vi "GetCommand.vi"(8 "error in (no error)":errorcluster, 11 "Controller in":refnum<class "Controller.lvclass">) -> (0 "error out":errorcluster, 3 "Controller out":refnum<class "Controller.lvclass">)   [LabVIEW 2014, in "Controller.lvclass"]
uses:
  Controller.lvclass
  <vilib>/Utility/inputDevices.llb/joystickAcquire.vi
panel:
  in  "DeviceType":refnum<k1>
  out "DeviceType":refnum<k1>
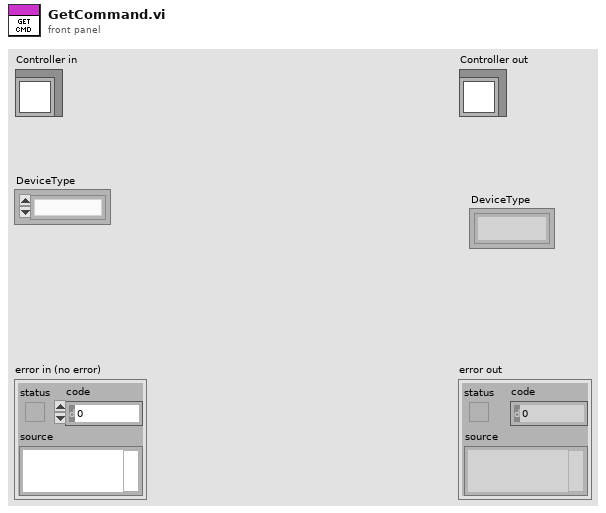
[diagram p1: front panel]
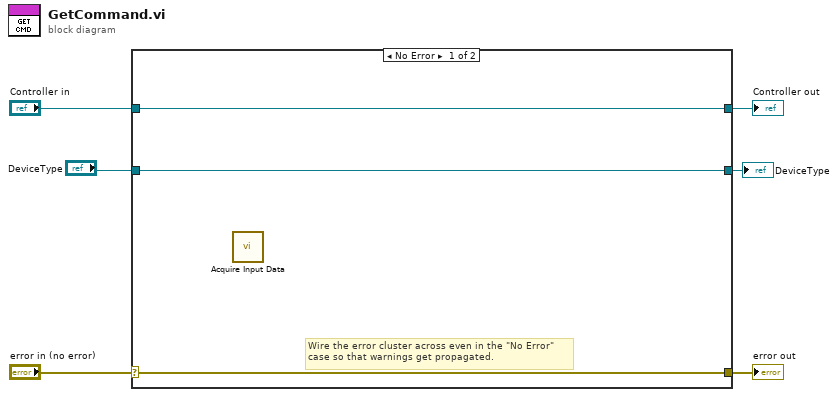
[diagram p0: block diagram]
diagram:
  n1 = case shown="No Error" "error in (no error)" {
    selector: "error in (no error)" -> [w8 w11]
    tunnel: [w8 w11] -> w5
    tunnel: [w9 w10] -> w3
    tunnel: "Controller in" -> [w9 w10]
    tunnel: "DeviceType" -> [w7 _]
    tunnel: [w7 _] -> w1
    frame No Error {
      # "Wire the error cluster across even in the \"No Error\"\ncase so that warnings get propagated."
      n2 = call-poly <vilib>:"Acquire Input Data.vi"() -> ()  [unwired: 15 in, 5 out]
    }
    frame Error {
    }
  }
  "error out" <- w5
  "Controller out" <- w3
  "DeviceType" <- w1
